vi "quizTres.vi"() -> ()   [LabVIEW 2020]
uses:
  <vilib>/Utility/file.llb/Read Delimited Spreadsheet (string).vi
  <vilib>/Utility/file.llb/Write Delimited Spreadsheet (string).vi
panel:
  in  "Numeric":i32
  in  "Boolean 2":bool
  in  "Boolean":bool
  in  "Sesion Usuario 2":enum32{"Inicio", "login", "admin", "usuario"}(tab) caption="Tab Control"
  in  "Iniciar 2":bool
  in  "Iniciar sesion 2":bool
  in  "Contraseña 2":string caption="Contraseña"
  in  "Usuario 2":string caption="Usuario"
  in  "Cerrar admin 2":bool
  in  "Eliminar 2":bool
  in  "Agregar 2":bool
  in  "Usuario nuevo2":string caption="Usuario nuevo"
  in  "Contraseña nueva 2":string caption="Contraseña nueva"
  in  "Usuario a eliminar2":string caption="Usuario a eliminar"
  out "Base de datos 2":string[][](array[string]) caption="BASE DE DATOS"
  in  "Cambio semaforo 2":u32 caption="Cambio semaforo"
  out "Semaforo verde 2":bool[][](array[boolean])
  out "Semaforo rojo 2":bool[][](array[boolean])
  in  "Silueta verde 2":bool[][](array[boolean])
  in  "Silueta rojo 2":bool[][](array[boolean])
  in  "Semaforo 2":bool
  in  "Cerrar usuario 2":bool
  in  "Sesion Usuario 1":enum32{"Inicio", "login", "admin", "usuario"}(tab) caption="Tab Control"
  in  "Iniciar 1":bool
  in  "Iniciar sesion 1":bool
  in  "Contraseña 1":string caption="Contraseña"
  in  "Usuario 1":string caption="Usuario"
  in  "Cerrar admin":bool
  in  "Eliminar 1":bool
  in  "Agregar 1":bool
  in  "Usuario nuevo 1":string caption="Usuario nuevo"
  in  "Contraseña nueva 1":string caption="Contraseña nueva"
  in  "Usuario a eliminar 1":string caption="Usuario a eliminar"
  out "Base de datos":string[][](array[string]) caption="BASE DE DATOS"
  in  "Cambio semaforo":u32
  out "Semaforo verde":bool[][](array[boolean])
  out "Semaforo rojo":bool[][](array[boolean])
  in  "Silueta verde":bool[][](array[boolean])
  in  "Silueta rojo":bool[][](array[boolean])
  in  "Semaforo 1":bool
  in  "Cerrar usuario":bool
  # "LOGIN"
  # "MENU DE ADMIN"
  # "AGREGAR USUARIOS"
  # "Usuario"
  # "Contraseña"
  # "ELIMINAR USUARIOS"
  # "MENU DE USUARIO"
  # "LOGIN"
  # "MENU DE ADMIN"
  # "AGREGAR USUARIOS"
  # "Usuario"
  # "Contraseña"
  # "ELIMINAR USUARIOS"
  # "MENU DE USUARIO"
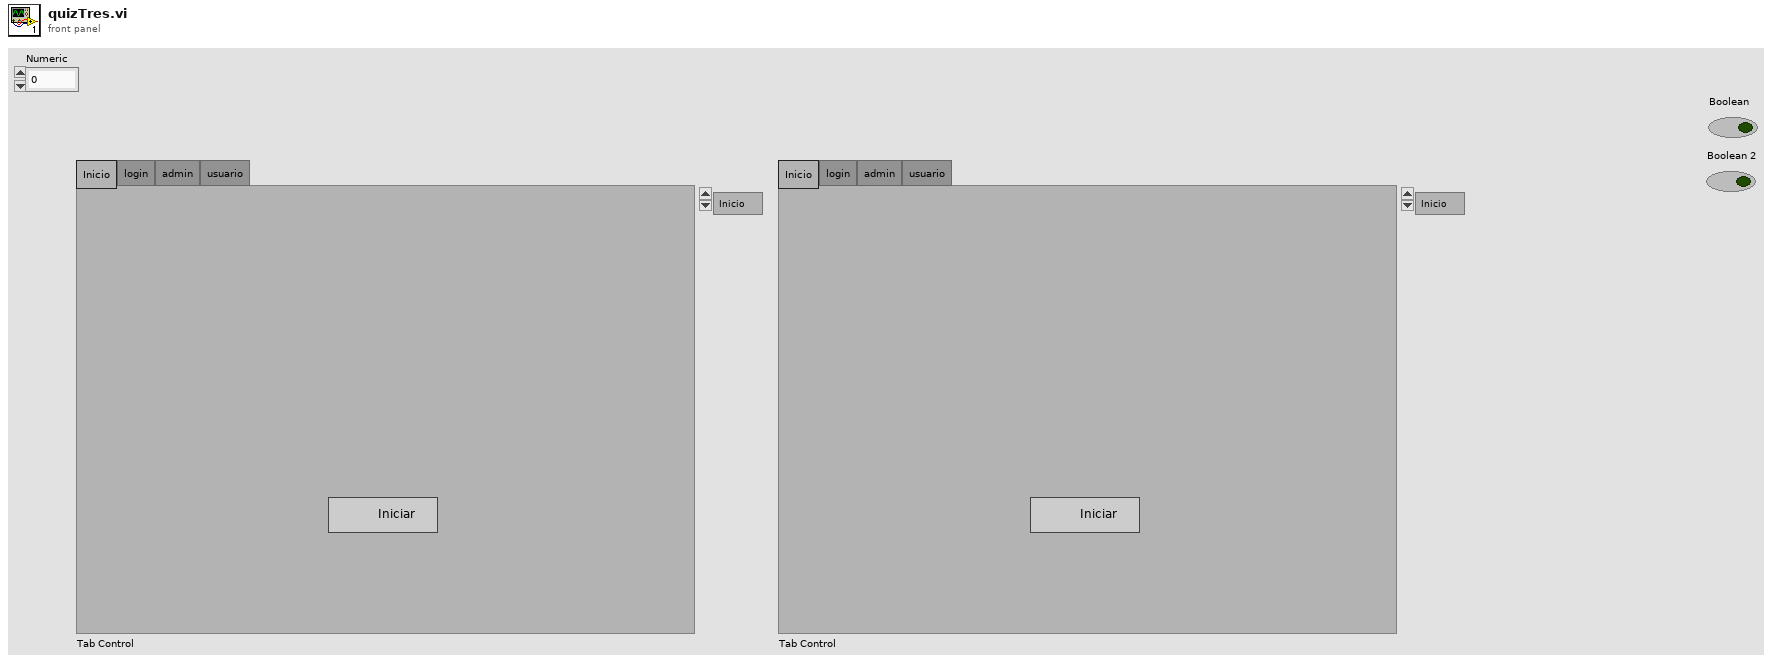
[diagram p1: front panel]
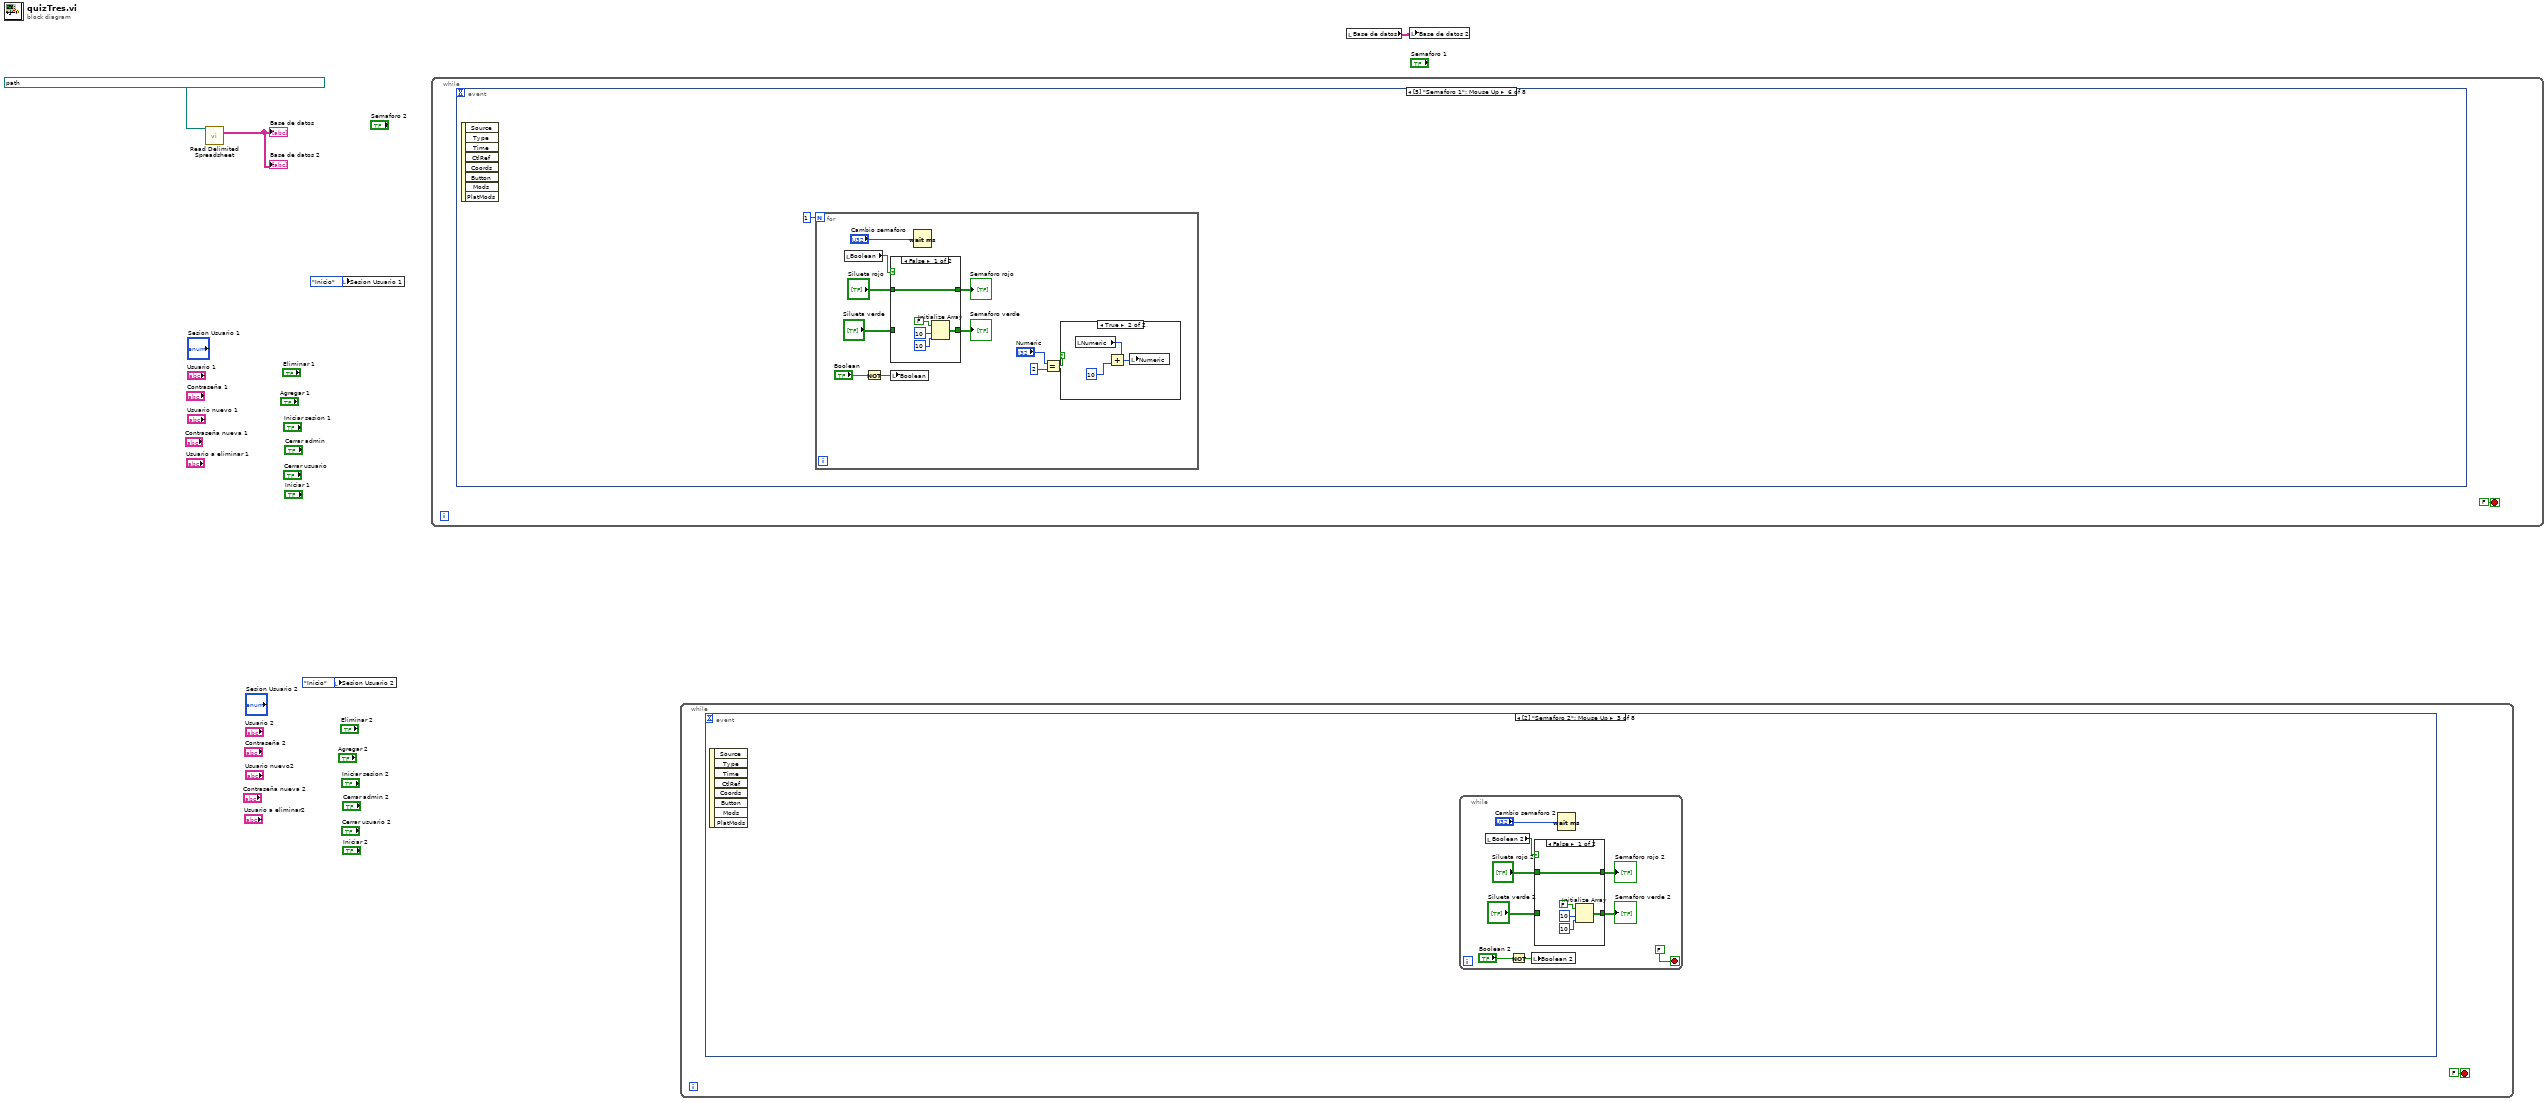
[diagram p0: block diagram]
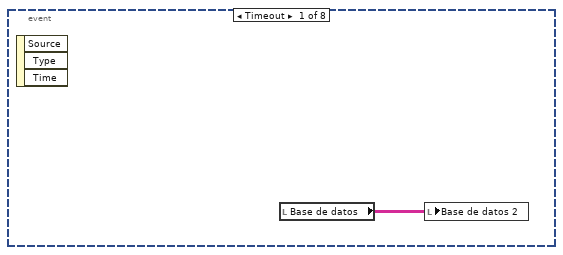
[diagram p2: hidden frame]
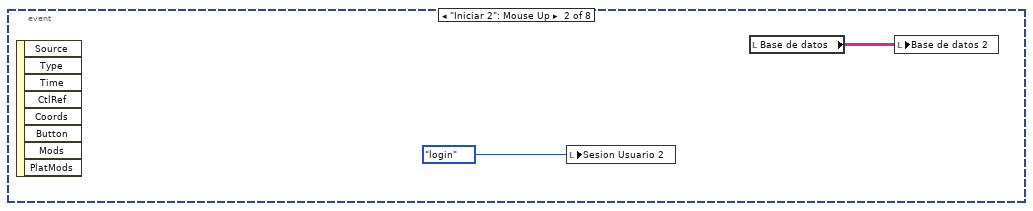
[diagram p3: hidden frame]
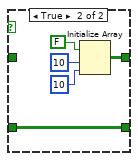
[diagram p4: hidden frame]
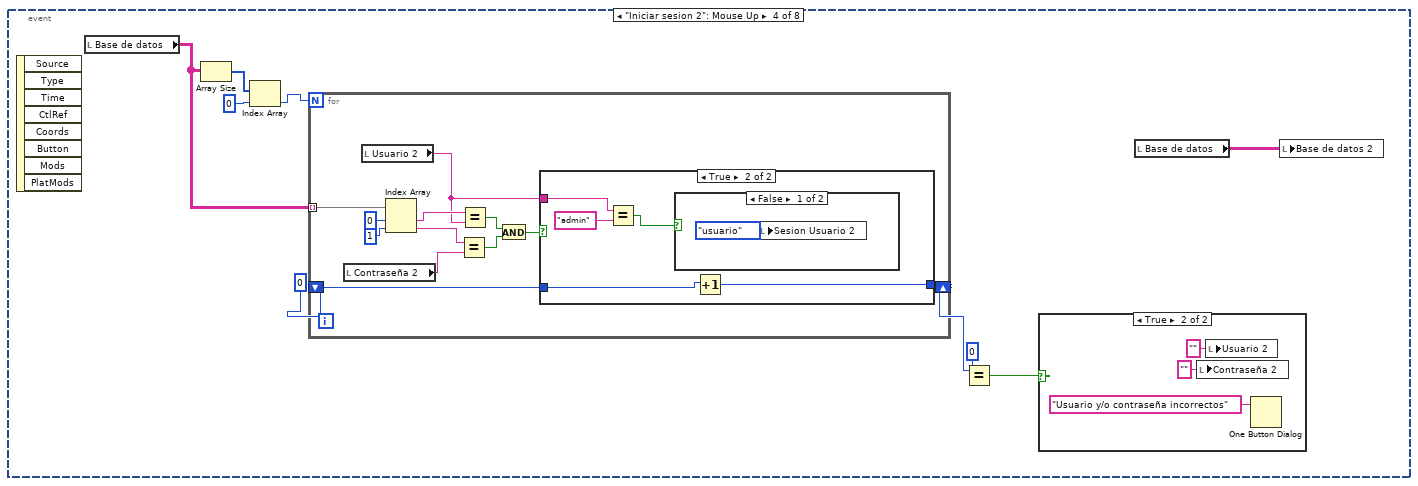
[diagram p5: hidden frame]
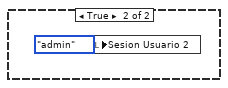
[diagram p8: hidden frame]
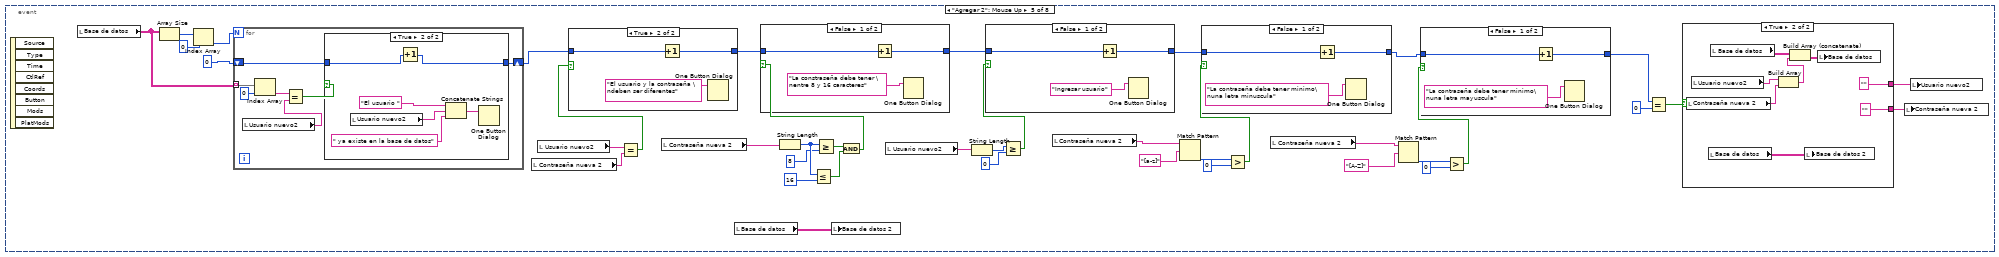
[diagram p9: hidden frame]
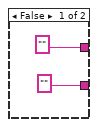
[diagram p10: hidden frame]
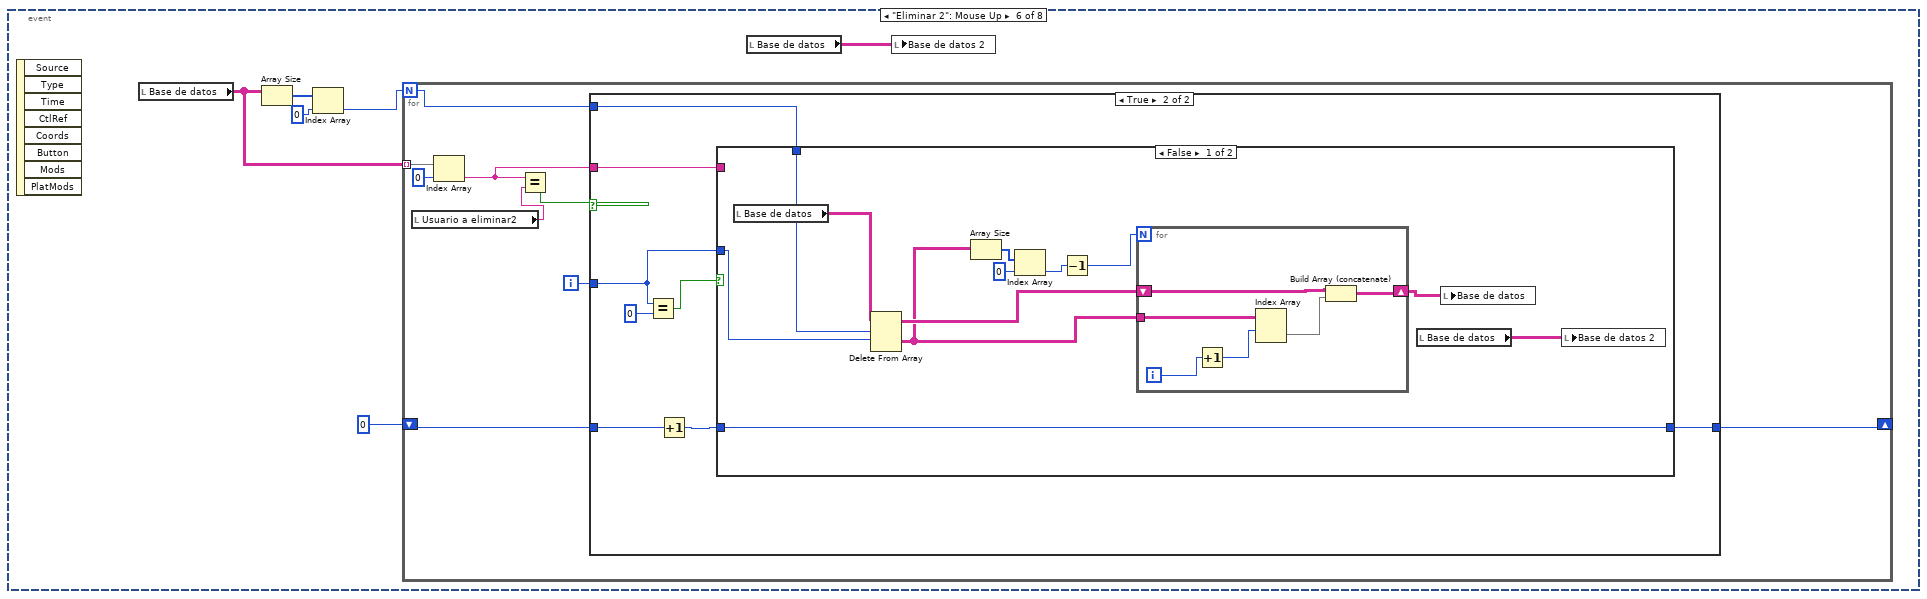
[diagram p17: hidden frame]
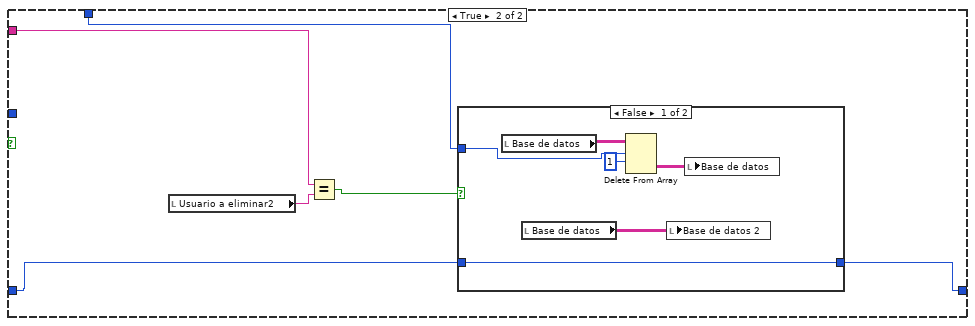
[diagram p19: hidden frame]
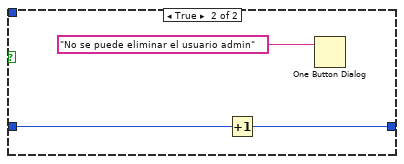
[diagram p20: hidden frame]
diagram:
  n1 = call-poly <vilib>:"Read Delimited Spreadsheet.vi"("file path (dialog if empty)"=path "C:/Users/Cristian/Desktop/Lenguaje de programación 2/Examen 3 Inicio de sesiones/Base de datos.txt") -> ("all rows"=→"Base de datos" →"Base de datos 2":string[][])  [unwired: 9 in, 5 out]
  n2 = local write "Sesion Usuario 2"(enum32{"Inicio", "login", "admin", "usuario"}."Inicio" ("Tab Control")) -> ()
  n3 = local write "Sesion Usuario 1"(enum32{"Inicio", "login", "admin", "usuario"}."Inicio" ("Tab Control")) -> ()
  n4 = while {
    stop <- FALSE stop-if-true
    n5 = event shown="[5] \"Semaforo 1\": Mouse Up" {
      selector: _ -> [_ _ _ _ _ _ _ _]
      dyn-events: _ -> [_ _ _ _ _ _ _ _]
      timeout: _ -> [_ _ _ _ _ _ _ _]
      event Timeout {
        n6 = event-data() -> ()  [unwired: 1 in, 3 out]
        n7 = local read "Base de datos"() -> (w8:string[][])
        n8 = call-poly <vilib>:"Write Delimited Spreadsheet.vi"("file path (dialog if empty)"=path "C:/Users/Cristian/Desktop/Lenguaje de programación 2/Examen 3 Inicio de sesiones/Base de datos.txt", "2D data"=w8) -> ()  [unwired: 12 in, 2 out]
        n9 = local read "Base de datos"() -> (w7:string[][])
        n10 = local write "Base de datos 2"(w7) -> ()
      }
      event "Iniciar 1": Mouse Up {
        n11 = event-data() -> ()  [unwired: 1 in, 8 out]
        n12 = local write "Sesion Usuario 1"(enum32{"Inicio", "login", "admin", "usuario"}."login" ("Tab Control")) -> ()
        n13 = local read "Base de datos"() -> (w10:string[][])
        n14 = local write "Base de datos 2"(w10) -> ()
      }
      event "Iniciar sesion 1": Mouse Up {
        n15 = event-data() -> ()  [unwired: 1 in, 8 out]
        n16 = local read "Base de datos"() -> (w17:string[][])
        n17 = Array Size(array=w17) -> (size(s)=w20:i32[])
        n18 = Index Array(array=w20, index=0) -> (element=w18:i32)
        n19 = for {
          N: w18 -> [_]
          tunnel: w17 -> [w35] mode=indexing
          shift-right: [w24] -> w14
          shift-left: 0 -> [w25]
          n20 = local read "Contraseña 1"() -> (w32:string)
          n21 = local read "Usuario 1"() -> (w26:string)
          n22 = Index Array "Index Array"(array=w35, index #1=0 ("index"), index #2=1 ("index")) -> (element #1=w30:string, element #2=w31:string)
          n23 = Equal?(x=w31, y=w32) -> (x = y?=w28:bool)
          n24 = Equal?(x=w30, y=w26) -> (x = y?=w29:bool)
          n25 = And(x=w29, y=w28) -> (x .and. y?=w27:bool)
          n26 = case shown="True" w27 {
            tunnel: w26 -> [_ w41]
            tunnel: w25 -> [w36 w38]
            tunnel: [w36 w37] -> w24
            frame False {
            }
            frame True {
              n27 = Equal?(x=w41, y="admin") -> (x = y?=w39:bool)
              n28 = case shown="False" w39 {
                frame False {
                  n29 = local write "Sesion Usuario 1"(enum32{"Inicio", "login", "admin", "usuario"}."usuario" ("Tab Control")) -> ()
                }
                frame True {
                  n30 = local write "Sesion Usuario 1"(enum32{"Inicio", "login", "admin", "usuario"}."admin" ("Tab Control")) -> ()
                }
              }
              n31 = Increment(x=w38) -> (x+1=w37:i32)
            }
          }
        }
        n32 = Equal?(x=w14, y=0) -> (x = y?=w15:bool)
        n33 = case shown="False" w15 {
          frame False {
          }
          frame True {
            n34 = local write "Contraseña 1"("" ("Contraseña")) -> ()
            n35 = local write "Usuario 1"("" ("Usuario")) -> ()
            n36 = One Button Dialog(message="Usuario y/o contraseña incorrectos") -> ()  [unwired: 1 in, 1 out]
          }
        }
        n37 = local read "Base de datos"() -> (w12:string[][])
        n38 = local write "Base de datos 2"(w12) -> ()
      }
      event "Agregar 1": Mouse Up {
        n39 = event-data() -> ()  [unwired: 1 in, 8 out]
        n40 = local read "Base de datos"() -> (w78:string[][])
        n41 = Array Size(array=w78) -> (size(s)=w82:i32[])
        n42 = Index Array(array=w82, index=0) -> (element=w80:i32)
        n43 = for {
          N: w80 -> [_]
          shift-right: [w113] -> w74
          shift-left: 0 ("index") -> [w114]
          tunnel: w78 -> [w119] mode=indexing
          n44 = local read "Usuario nuevo 1"() -> (w116:string)
          n45 = Index Array(array=w119, index=0) -> (element=w117:string)
          n46 = Equal?(x=w117, y=w116) -> (x = y?=w115:bool)
          n47 = case shown="True" w115 {
            tunnel: w114 -> [w120 w126]
            tunnel: [w120 w125] -> w113
            frame False {
            }
            frame True {
              n48 = local read "Usuario nuevo 1"() -> (w123:string)
              n49 = Increment(x=w126) -> (x+1=w125:i32)
              n50 = Concatenate Strings("El usuario " ("string"), w123, " ya existe en la base de datos" ("string")) -> (w121:string)
              n51 = One Button Dialog(message=w121) -> ()  [unwired: 1 in, 1 out]
            }
          }
        }
        n52 = local read "Contraseña nueva 1"() -> (w76:string)
        n53 = local read "Usuario nuevo 1"() -> (w77:string)
        n54 = Equal?(x=w77, y=w76) -> (x = y?=w75:bool)
        n55 = case shown="True" w75 {
          tunnel: w74 -> [w109 w112]
          tunnel: [w109 w111] -> w66
          frame False {
          }
          frame True {
            n56 = Increment(x=w112) -> (x+1=w111:i32)
            n57 = One Button Dialog(message="El usuario y la contraseña \ndeben ser diferentes") -> ()  [unwired: 1 in, 1 out]
          }
        }
        n58 = local read "Contraseña nueva 1"() -> (w73:string)
        n59 = String Length(string=w73) -> (length=w72:i32)
        n60 = Less Or Equal?(x=w72, y=16) -> (x <= y?=w68:bool)
        n61 = Greater Or Equal?(x=w72, y=8) -> (x >= y?=w69:bool)
        n62 = And(x=w69, y=w68) -> (x .and. y?=w67:bool)
        n63 = case shown="False" w67 {
          tunnel: w66 -> [w107 w108]
          tunnel: [w106 w108] -> w62
          frame False {
            n64 = Increment(x=w107) -> (x+1=w106:i32)
            n65 = One Button Dialog(message="La constraseña debe tener \nentre 8 y 16 caracteres") -> ()  [unwired: 1 in, 1 out]
          }
          frame True {
          }
        }
        n66 = local read "Usuario nuevo 1"() -> (w64:string)
        n67 = String Length(string=w64) -> (length=w65:i32)
        n68 = Greater Or Equal?(x=w65, y=0) -> (x >= y?=w61:bool)
        n69 = case shown="False" w61 {
          tunnel: w62 -> [w103 w104]
          tunnel: [w102 w104] -> w55
          frame False {
            n70 = Increment(x=w103) -> (x+1=w102:i32)
            n71 = One Button Dialog(message="Ingresar usuario") -> ()  [unwired: 1 in, 1 out]
          }
          frame True {
          }
        }
        n72 = local read "Contraseña nueva 1"() -> (w60:string)
        n73 = Match Pattern(string=w60, regular expression="[a-z]") -> (offset past match=w58:i32)  [unwired: 1 in, 3 out]
        n74 = Greater?(x=w58, y=0) -> (0:w56:bool)
        n75 = case shown="False" w56 {
          tunnel: w55 -> [w99 w100]
          tunnel: [w98 w100] -> w49
          frame False {
            n76 = Increment(x=w99) -> (x+1=w98:i32)
            n77 = One Button Dialog(message="La contraseña debe tener minimo\nuna letra minuscula") -> ()  [unwired: 1 in, 1 out]
          }
          frame True {
          }
        }
        n78 = local read "Contraseña nueva 1"() -> (w51:string)
        n79 = Match Pattern(string=w51, regular expression="[A-Z]") -> (offset past match=w52:i32)  [unwired: 1 in, 3 out]
        n80 = Greater?(x=w52, y=0) -> (0:w54:bool)
        n81 = case shown="False" w54 {
          tunnel: w49 -> [w95 w96]
          tunnel: [w94 w96] -> w48
          frame False {
            n82 = Increment(x=w95) -> (x+1=w94:i32)
            n83 = One Button Dialog(message="La contraseña debe tener minimo\nuna letra mayuscula") -> ()  [unwired: 1 in, 1 out]
          }
          frame True {
          }
        }
        n84 = Equal?(x=w48, y=0) -> (x = y?=w46:bool)
        n85 = case shown="True" w46 {
          tunnel: ["" ("Usuario nuevo 1") "" ("Usuario nuevo 1")] -> w45
          tunnel: ["" ("Usuario nuevo 1") "" ("Usuario nuevo 1")] -> w44
          frame False {
          }
          frame True {
            n86 = local read "Contraseña nueva 1"() -> (w90:string)
            n87 = local read "Usuario nuevo 1"() -> (w91:string)
            n88 = local read "Base de datos"() -> (w92:string[][])
            n89 = local read "Base de datos"() -> (w85:string[][])
            n90 = Build Array(w91, w90) -> (w89:string[])
            n91 = Build Array (concatenate)(w92, w89) -> (w88:string[][])
            n92 = local write "Base de datos 2"(w85) -> ()
            n93 = local write "Base de datos"(w88) -> ()
          }
        }
        n94 = local write "Contraseña nueva 1"(w44) -> ()
        n95 = local write "Usuario nuevo 1"(w45) -> ()
      }
      event "Eliminar 1": Mouse Up {
        n96 = event-data() -> ()  [unwired: 1 in, 8 out]
        n97 = local read "Base de datos"() -> (w128:string[][])
        n98 = Array Size(array=w128) -> (size(s)=w131:i32[])
        n99 = Index Array(array=w131, index=0) -> (element=w129:i32)
        n100 = for {
          N: w129 -> [w136]
          tunnel: w128 -> [w140] mode=indexing
          shift-right: [w133] -> _
          shift-left: 0 ("y") -> [w134]
          i -> [w135]
          n101 = local read "Usuario a eliminar 1"() -> (w138:string)
          n102 = Index Array(array=w140, index=0) -> (element=w132:string)
          n103 = Equal?(x=w132, y=w138) -> (x = y?=w137:bool)
          n104 = case shown="True" w137 {
            tunnel: w136 -> [_ w149]
            tunnel: w135 -> [_ w146]
            tunnel: w134 -> [w141 w145]
            tunnel: [w141 w143] -> w133
            tunnel: w132 -> [_ w142]
            frame False {
            }
            frame True {
              n105 = Equal?(x=w146, y=0) -> (x = y?=w147:bool)
              n106 = Increment(x=w145) -> (x+1=w144:i32)
              n107 = case shown="False" w147 {
                tunnel: w149 -> [w160 w168]
                tunnel: w146 -> [w159 _]
                tunnel: w144 -> [w158 w170]
                tunnel: [w158 w169] -> w143
                tunnel: w142 -> [_ w173]
                frame False {
                  n108 = local read "Base de datos"() -> (w157:string[][])
                  n109 = Delete From Array(array=w157, length=w160, index (row)=w159) -> (deleted portion=w151:string[][], array with subset deleted=w152:string[][])  [unwired: 1 in]
                  n110 = Array Size(array=w151) -> (size(s)=w156:i32[])
                  n111 = Index Array(array=w156, index=0) -> (element=w154:i32)
                  n112 = Decrement(x=w154) -> (x-1=w153:i32)
                  n113 = for {
                    N: w153 -> [_]
                    shift-right: [w162] -> w150
                    shift-left: w152 -> [w164]
                    tunnel: w151 -> [w165]
                    i -> [w167]
                    n114 = Increment(x=w167) -> (x+1=w166:i32)
                    n115 = local read "Base de datos"() -> (w161:string[][])
                    n116 = Index Array(array=w165, index (row)=w166) -> (element=w163:string[])  [unwired: 1 in]
                    n117 = Build Array (concatenate)(w164, w163) -> (w162:string[][])
                    n118 = local write "Base de datos 2"(w161) -> ()
                  }
                  n119 = local write "Base de datos"(w150) -> ()
                }
                frame True {
                  n120 = local read "Usuario a eliminar 1"() -> (w172:string)
                  n121 = Equal?(x=w173, y=w172) -> (x = y?=w171:bool)
                  n122 = case shown="True" w171 {
                    tunnel: w170 -> [w175 w182]
                    tunnel: [w175 w181] -> w169
                    tunnel: w168 -> [w178 _]
                    frame False {
                      n123 = local read "Base de datos"() -> (w179:string[][])
                      n124 = local read "Base de datos"() -> (w174:string[][])
                      n125 = Delete From Array(array=w179, length=w178, index (row)=1) -> (deleted portion=w176:string[][])  [unwired: 1 in, 1 out]
                      n126 = local write "Base de datos 2"(w174) -> ()
                      n127 = local write "Base de datos"(w176) -> ()
                    }
                    frame True {
                      n128 = Increment(x=w182) -> (x+1=w181:i32)
                      n129 = One Button Dialog(message="No se puede eliminar el usuario admin") -> ()  [unwired: 1 in, 1 out]
                    }
                  }
                }
              }
            }
          }
        }
      }
      event "Semaforo 1": Mouse Up {
        n130 = event-data() -> ()  [unwired: 1 in, 8 out]
        n131 = for {
          N: 1 -> [_]
          n132 = local read "Boolean"() -> (w189:bool)
          n133 = Not(x="Boolean") -> (.not. x?=w192:bool)
          n134 = case shown="False" w189 {
            tunnel: "Silueta verde" -> [_ w207]
            tunnel: [w198 w207] -> w188
            tunnel: "Silueta rojo" -> [w202 _]
            tunnel: [w202 w203] -> w187
            frame False {
              n135 = Initialize Array(FALSE, 10 ("dimension size"), 10 ("dimension size")) -> (w198:bool[][])
            }
            frame True {
              n136 = Initialize Array(FALSE, 10 ("dimension size"), 10 ("dimension size")) -> (w203:bool[][])
            }
          }
          "Semaforo verde" <- w188
          "Semaforo rojo" <- w187
          n137 = local write "Boolean"(w192) -> ()
          n138 = Wait (ms)(milliseconds to wait="Cambio semaforo") -> ()  [unwired: 1 out]
          n139 = Equal?(x="Numeric", y=2) -> (x = y?=w184:bool)
          n140 = case shown="True" w184 {
            frame False {
            }
            frame True {
              n141 = local read "Numeric"() -> (w197:i32)
              n142 = Add(x=w197, y=10) -> (x+y=w195:i32)
              n143 = local write "Numeric"(w195) -> ()
            }
          }
        }
      }
      event "Cerrar admin": Mouse Up {
        n144 = event-data() -> ()  [unwired: 1 in, 8 out]
        n145 = local write "Sesion Usuario 1"(enum32{"Inicio", "login", "admin", "usuario"}."login" ("Tab Control")) -> ()
        n146 = local write "Usuario 1"("" ("Usuario 1")) -> ()
        n147 = local write "Contraseña 1"("" ("Contraseña 1")) -> ()
        n148 = local read "Base de datos"() -> (w208:string[][])
        n149 = local write "Base de datos 2"(w208) -> ()
      }
      event "Cerrar usuario": Mouse Up {
        n150 = event-data() -> ()  [unwired: 1 in, 8 out]
        n151 = local write "Usuario 1"("" ("Usuario 1")) -> ()
        n152 = local write "Sesion Usuario 1"(enum32{"Inicio", "login", "admin", "usuario"}."login" ("Tab Control")) -> ()
        n153 = local write "Contraseña 1"("" ("Contraseña 1")) -> ()
        n154 = local read "Base de datos"() -> (w212:string[][])
        n155 = local write "Base de datos 2"(w212) -> ()
      }
    }
  }
  n156 = while {
    stop <- FALSE stop-if-true
    n157 = event shown="[2] \"Semaforo 2\": Mouse Up" {
      selector: _ -> [_ _ _ _ _ _ _ _]
      dyn-events: _ -> [_ _ _ _ _ _ _ _]
      timeout: _ -> [_ _ _ _ _ _ _ _]
      event Timeout {
        n158 = event-data() -> ()  [unwired: 1 in, 3 out]
        n159 = local read "Base de datos"() -> (w217:string[][])
        n160 = local write "Base de datos 2"(w217) -> ()
      }
      event "Iniciar 2": Mouse Up {
        n161 = event-data() -> ()  [unwired: 1 in, 8 out]
        n162 = local write "Sesion Usuario 2"(enum32{"Inicio", "login", "admin", "usuario"}."login" ("Tab Control")) -> ()
        n163 = local read "Base de datos"() -> (w218:string[][])
        n164 = local write "Base de datos 2"(w218) -> ()
      }
      event "Semaforo 2": Mouse Up {
        n165 = event-data() -> ()  [unwired: 1 in, 8 out]
        n166 = while {
          stop <- FALSE stop-if-true
          n167 = local read "Boolean 2"() -> (w222:bool)
          n168 = Not(x="Boolean 2") -> (.not. x?=w226:bool)
          n169 = local write "Boolean 2"(w226) -> ()
          n170 = case shown="False" w222 {
            tunnel: "Silueta verde 2" -> [_ w238]
            tunnel: [w229 w238] -> w221
            tunnel: "Silueta rojo 2" -> [w233 _]
            tunnel: [w233 w234] -> w220
            frame False {
              n171 = Initialize Array(FALSE, 10 ("dimension size"), 10 ("dimension size")) -> (w229:bool[][])
            }
            frame True {
              n172 = Initialize Array(FALSE, 10 ("dimension size"), 10 ("dimension size")) -> (w234:bool[][])
            }
          }
          "Semaforo verde 2" <- w221
          "Semaforo rojo 2" <- w220
          n173 = Wait (ms)(milliseconds to wait="Cambio semaforo 2") -> ()  [unwired: 1 out]
        }
      }
      event "Iniciar sesion 2": Mouse Up {
        n174 = event-data() -> ()  [unwired: 1 in, 8 out]
        n175 = local read "Base de datos"() -> (w244:string[][])
        n176 = Array Size(array=w244) -> (size(s)=w247:i32[])
        n177 = Index Array(array=w247, index=0) -> (element=w245:i32)
        n178 = for {
          N: w245 -> [_]
          tunnel: w244 -> [w262] mode=indexing
          shift-right: [w251] -> w241
          shift-left: 0 -> [w252]
          n179 = local read "Contraseña 2"() -> (w259:string)
          n180 = local read "Usuario 2"() -> (w253:string)
          n181 = Index Array "Index Array"(array=w262, index #1=0 ("index"), index #2=1 ("index")) -> (element #1=w257:string, element #2=w258:string)
          n182 = Equal?(x=w258, y=w259) -> (x = y?=w255:bool)
          n183 = Equal?(x=w257, y=w253) -> (x = y?=w256:bool)
          n184 = And(x=w256, y=w255) -> (x .and. y?=w254:bool)
          n185 = case shown="True" w254 {
            tunnel: w253 -> [_ w268]
            tunnel: w252 -> [w263 w265]
            tunnel: [w263 w264] -> w251
            frame False {
            }
            frame True {
              n186 = Equal?(x=w268, y="admin") -> (x = y?=w266:bool)
              n187 = case shown="False" w266 {
                frame False {
                  n188 = local write "Sesion Usuario 2"(enum32{"Inicio", "login", "admin", "usuario"}."usuario" ("Tab Control")) -> ()
                }
                frame True {
                  n189 = local write "Sesion Usuario 2"(enum32{"Inicio", "login", "admin", "usuario"}."admin" ("Tab Control")) -> ()
                }
              }
              n190 = Increment(x=w265) -> (x+1=w264:i32)
            }
          }
        }
        n191 = Equal?(x=w241, y=0) -> (x = y?=w242:bool)
        n192 = case shown="True" w242 {
          frame False {
          }
          frame True {
            n193 = local write "Contraseña 2"("" ("Contraseña")) -> ()
            n194 = local write "Usuario 2"("" ("Usuario")) -> ()
            n195 = One Button Dialog(message="Usuario y/o contraseña incorrectos") -> ()  [unwired: 1 in, 1 out]
          }
        }
        n196 = local read "Base de datos"() -> (w239:string[][])
        n197 = local write "Base de datos 2"(w239) -> ()
      }
      event "Agregar 2": Mouse Up {
        n198 = event-data() -> ()  [unwired: 1 in, 8 out]
        n199 = local read "Base de datos"() -> (w306:string[][])
        n200 = Array Size(array=w306) -> (size(s)=w310:i32[])
        n201 = Index Array(array=w310, index=0) -> (element=w308:i32)
        n202 = for {
          N: w308 -> [_]
          shift-right: [w341] -> w302
          shift-left: 0 ("index") -> [w342]
          tunnel: w306 -> [w347] mode=indexing
          n203 = local read "Usuario nuevo2"() -> (w344:string)
          n204 = Index Array(array=w347, index=0) -> (element=w345:string)
          n205 = Equal?(x=w345, y=w344) -> (x = y?=w343:bool)
          n206 = case shown="True" w343 {
            tunnel: w342 -> [w348 w354]
            tunnel: [w348 w353] -> w341
            frame False {
            }
            frame True {
              n207 = local read "Usuario nuevo2"() -> (w351:string)
              n208 = Increment(x=w354) -> (x+1=w353:i32)
              n209 = Concatenate Strings("El usuario " ("string"), w351, " ya existe en la base de datos" ("string")) -> (w349:string)
              n210 = One Button Dialog(message=w349) -> ()  [unwired: 1 in, 1 out]
            }
          }
        }
        n211 = local read "Contraseña nueva 2"() -> (w304:string)
        n212 = local read "Usuario nuevo2"() -> (w305:string)
        n213 = Equal?(x=w305, y=w304) -> (x = y?=w303:bool)
        n214 = case shown="True" w303 {
          tunnel: w302 -> [w337 w340]
          tunnel: [w337 w339] -> w294
          frame False {
          }
          frame True {
            n215 = Increment(x=w340) -> (x+1=w339:i32)
            n216 = One Button Dialog(message="El usuario y la contraseña \ndeben ser diferentes") -> ()  [unwired: 1 in, 1 out]
          }
        }
        n217 = local read "Contraseña nueva 2"() -> (w301:string)
        n218 = local read "Base de datos"() -> (w271:string[][])
        n219 = String Length(string=w301) -> (length=w300:i32)
        n220 = Less Or Equal?(x=w300, y=16) -> (x <= y?=w296:bool)
        n221 = Greater Or Equal?(x=w300, y=8) -> (x >= y?=w297:bool)
        n222 = local write "Base de datos 2"(w271) -> ()
        n223 = And(x=w297, y=w296) -> (x .and. y?=w295:bool)
        n224 = case shown="False" w295 {
          tunnel: w294 -> [w335 w336]
          tunnel: [w334 w336] -> w290
          frame False {
            n225 = Increment(x=w335) -> (x+1=w334:i32)
            n226 = One Button Dialog(message="La constraseña debe tener \nentre 8 y 16 caracteres") -> ()  [unwired: 1 in, 1 out]
          }
          frame True {
          }
        }
        n227 = local read "Usuario nuevo2"() -> (w292:string)
        n228 = String Length(string=w292) -> (length=w293:i32)
        n229 = Greater Or Equal?(x=w293, y=0) -> (x >= y?=w289:bool)
        n230 = case shown="False" w289 {
          tunnel: w290 -> [w331 w332]
          tunnel: [w330 w332] -> w283
          frame False {
            n231 = Increment(x=w331) -> (x+1=w330:i32)
            n232 = One Button Dialog(message="Ingresar usuario") -> ()  [unwired: 1 in, 1 out]
          }
          frame True {
          }
        }
        n233 = local read "Contraseña nueva 2"() -> (w288:string)
        n234 = Match Pattern(string=w288, regular expression="[a-z]") -> (offset past match=w286:i32)  [unwired: 1 in, 3 out]
        n235 = Greater?(x=w286, y=0) -> (0:w284:bool)
        n236 = case shown="False" w284 {
          tunnel: w283 -> [w327 w328]
          tunnel: [w326 w328] -> w277
          frame False {
            n237 = Increment(x=w327) -> (x+1=w326:i32)
            n238 = One Button Dialog(message="La contraseña debe tener minimo\nuna letra minuscula") -> ()  [unwired: 1 in, 1 out]
          }
          frame True {
          }
        }
        n239 = local read "Contraseña nueva 2"() -> (w279:string)
        n240 = Match Pattern(string=w279, regular expression="[A-Z]") -> (offset past match=w280:i32)  [unwired: 1 in, 3 out]
        n241 = Greater?(x=w280, y=0) -> (0:w282:bool)
        n242 = case shown="False" w282 {
          tunnel: w277 -> [w323 w324]
          tunnel: [w322 w324] -> w276
          frame False {
            n243 = Increment(x=w323) -> (x+1=w322:i32)
            n244 = One Button Dialog(message="La contraseña debe tener minimo\nuna letra mayuscula") -> ()  [unwired: 1 in, 1 out]
          }
          frame True {
          }
        }
        n245 = Equal?(x=w276, y=0) -> (x = y?=w274:bool)
        n246 = case shown="True" w274 {
          tunnel: ["" ("Usuario nuevo 1") "" ("Usuario nuevo 1")] -> w273
          tunnel: ["" ("Usuario nuevo 1") "" ("Usuario nuevo 1")] -> w272
          frame False {
          }
          frame True {
            n247 = local read "Contraseña nueva 2"() -> (w318:string)
            n248 = local read "Usuario nuevo2"() -> (w319:string)
            n249 = local read "Base de datos"() -> (w313:string[][])
            n250 = local read "Base de datos"() -> (w320:string[][])
            n251 = Build Array(w319, w318) -> (w317:string[])
            n252 = Build Array (concatenate)(w320, w317) -> (w316:string[][])
            n253 = local write "Base de datos 2"(w313) -> ()
            n254 = local write "Base de datos"(w316) -> ()
          }
        }
        n255 = local write "Contraseña nueva 2"(w272) -> ()
        n256 = local write "Usuario nuevo2"(w273) -> ()
      }
      event "Eliminar 2": Mouse Up {
        n257 = event-data() -> ()  [unwired: 1 in, 8 out]
        n258 = local read "Base de datos"() -> (w357:string[][])
        n259 = Array Size(array=w357) -> (size(s)=w360:i32[])
        n260 = Index Array(array=w360, index=0) -> (element=w358:i32)
        n261 = for {
          N: w358 -> [w365]
          tunnel: w357 -> [w369] mode=indexing
          shift-right: [w362] -> _
          shift-left: 0 ("y") -> [w363]
          i -> [w364]
          n262 = local read "Usuario a eliminar2"() -> (w367:string)
          n263 = Index Array(array=w369, index=0) -> (element=w361:string)
          n264 = Equal?(x=w361, y=w367) -> (x = y?=w366:bool)
          n265 = case shown="True" w366 {
            tunnel: w365 -> [_ w378]
            tunnel: w364 -> [_ w375]
            tunnel: w363 -> [w370 w374]
            tunnel: [w370 w372] -> w362
            tunnel: w361 -> [_ w371]
            frame False {
            }
            frame True {
              n266 = Equal?(x=w375, y=0) -> (x = y?=w376:bool)
              n267 = Increment(x=w374) -> (x+1=w373:i32)
              n268 = case shown="False" w376 {
                tunnel: w378 -> [w390 w397]
                tunnel: w375 -> [w389 _]
                tunnel: w373 -> [w388 w399]
                tunnel: [w388 w398] -> w372
                tunnel: w371 -> [_ w402]
                frame False {
                  n269 = local read "Base de datos"() -> (w387:string[][])
                  n270 = Delete From Array(array=w387, length=w390, index (row)=w389) -> (deleted portion=w381:string[][], array with subset deleted=w382:string[][])  [unwired: 1 in]
                  n271 = Array Size(array=w381) -> (size(s)=w386:i32[])
                  n272 = Index Array(array=w386, index=0) -> (element=w384:i32)
                  n273 = Decrement(x=w384) -> (x-1=w383:i32)
                  n274 = for {
                    N: w383 -> [_]
                    shift-right: [w391] -> w380
                    shift-left: w382 -> [w393]
                    tunnel: w381 -> [w394]
                    i -> [w396]
                    n275 = Increment(x=w396) -> (x+1=w395:i32)
                    n276 = Index Array(array=w394, index (row)=w395) -> (element=w392:string[])  [unwired: 1 in]
                    n277 = Build Array (concatenate)(w393, w392) -> (w391:string[][])
                  }
                  n278 = local read "Base de datos"() -> (w379:string[][])
                  n279 = local write "Base de datos"(w380) -> ()
                  n280 = local write "Base de datos 2"(w379) -> ()
                }
                frame True {
                  n281 = local read "Usuario a eliminar2"() -> (w401:string)
                  n282 = Equal?(x=w402, y=w401) -> (x = y?=w400:bool)
                  n283 = case shown="False" w400 {
                    tunnel: w399 -> [w404 w411]
                    tunnel: [w404 w410] -> w398
                    tunnel: w397 -> [w407 _]
                    frame False {
                      n284 = local read "Base de datos"() -> (w408:string[][])
                      n285 = local read "Base de datos"() -> (w403:string[][])
                      n286 = Delete From Array(array=w408, length=w407, index (row)=1) -> (deleted portion=w405:string[][])  [unwired: 1 in, 1 out]
                      n287 = local write "Base de datos 2"(w403) -> ()
                      n288 = local write "Base de datos"(w405) -> ()
                    }
                    frame True {
                      n289 = Increment(x=w411) -> (x+1=w410:i32)
                      n290 = One Button Dialog(message="No se puede eliminar el usuario admin") -> ()  [unwired: 1 in, 1 out]
                    }
                  }
                }
              }
            }
          }
        }
        n291 = local read "Base de datos"() -> (w355:string[][])
        n292 = local write "Base de datos 2"(w355) -> ()
      }
      event "Cerrar admin 2": Mouse Up {
        n293 = event-data() -> ()  [unwired: 1 in, 8 out]
        n294 = local write "Sesion Usuario 2"(enum32{"Inicio", "login", "admin", "usuario"}."login" ("Tab Control")) -> ()
        n295 = local write "Usuario 2"("" ("Usuario 1")) -> ()
        n296 = local write "Contraseña 2"("" ("Contraseña 1")) -> ()
        n297 = local read "Base de datos"() -> (w412:string[][])
        n298 = local write "Base de datos 2"(w412) -> ()
      }
      event "Cerrar usuario 2": Mouse Up {
        n299 = event-data() -> ()  [unwired: 1 in, 8 out]
        n300 = local write "Usuario 2"("" ("Usuario 1")) -> ()
        n301 = local write "Contraseña 2"("" ("Contraseña 1")) -> ()
        n302 = local write "Sesion Usuario 2"(enum32{"Inicio", "login", "admin", "usuario"}."login" ("Tab Control")) -> ()
        n303 = local read "Base de datos"() -> (w416:string[][])
        n304 = local write "Base de datos 2"(w416) -> ()
      }
    }
  }
  n305 = local read "Base de datos"() -> (w1:string[][])
  n306 = local write "Base de datos 2"(w1) -> ()
